vi "Stop Digital Audio Generation.vi"(8 "error in (no error)":errorcluster, 11 "PCM tasks":T2) -> (0 "error out":errorcluster)   [LabVIEW 2021]
uses:
  <vilib>/PDM Acquisition Toolkit/host/API/PDM Acquisition Toolkit.lvlib
  <vilib>/PDM Acquisition Toolkit/host/Classes/Tasks/PCM Output/PCM Output Task.lvclass
  <vilib>/PDM Acquisition Toolkit/host/Classes/Tasks/PCM Output/Controls/PCM Output Task DVR.ctl
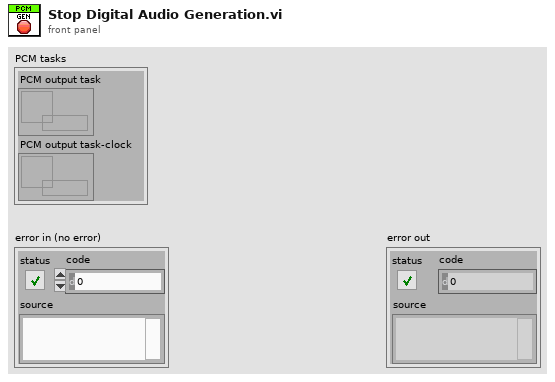
[diagram p1: front panel]
types:
  T1 = typedef "PDM Acquisition Class Library.lvlib/PCM Output Task.lvclass/PCM Output Task DVR.ctl" = refnum<data-value>
  T2 = cluster{"PCM output task":T1, "PCM output task-clock":T1}
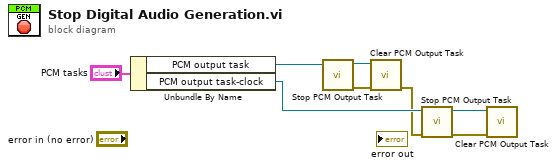
[diagram p0: block diagram]
diagram:
  n1 = Unbundle By Name("PCM tasks") -> ("PCM output task"=w6:T1, "PCM output task-clock"=w7:T1)
  n2 = call <vilib>:"Stop PCM Output Task.vi"("PCM output task In"=w6) -> ("error out"=w5:errorcluster, "PCM output task out"=w4:T1)  [unwired: 9 in]
  n3 = call <vilib>:"Clear PCM Output Task.vi"("error in"=w5, "PCM output task in"=w4) -> ("error out"=w1:errorcluster)  [unwired: 9 in]
  n4 = call <vilib>:"Stop PCM Output Task.vi"("error in"=w1, "PCM output task In"=w7) -> ("error out"=w3:errorcluster, "PCM output task out"=w2:T1)  [unwired: 8 in]
  n5 = call <vilib>:"Clear PCM Output Task.vi"("error in"=w3, "PCM output task in"=w2) -> ()  [unwired: 9 in, 1 out]
